vi "Directory handler.vi"() -> ()   [LabVIEW 2011]
panel:
  in  "Type of Files (*.csv; *.txt)":string="Select the Loc"
  in  "Prompt for Directory Diolog":string="Select the Loc"
  out "error in (no error) 2":errorcluster
  out "Path output":path
  in  "Start Path":path
  in  "error in (no error)":errorcluster
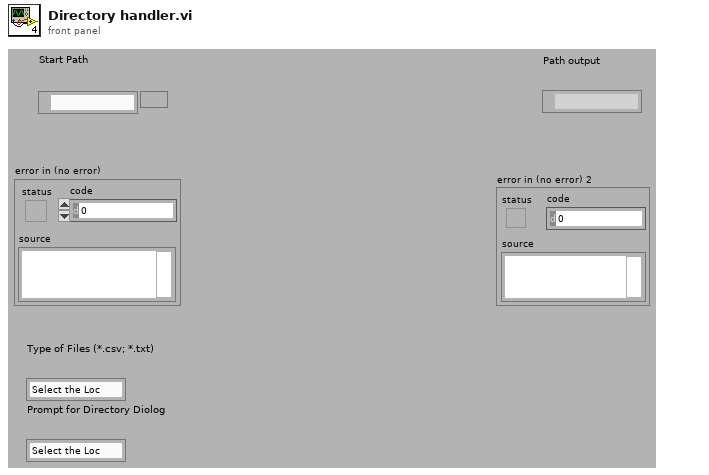
[diagram p1: front panel]
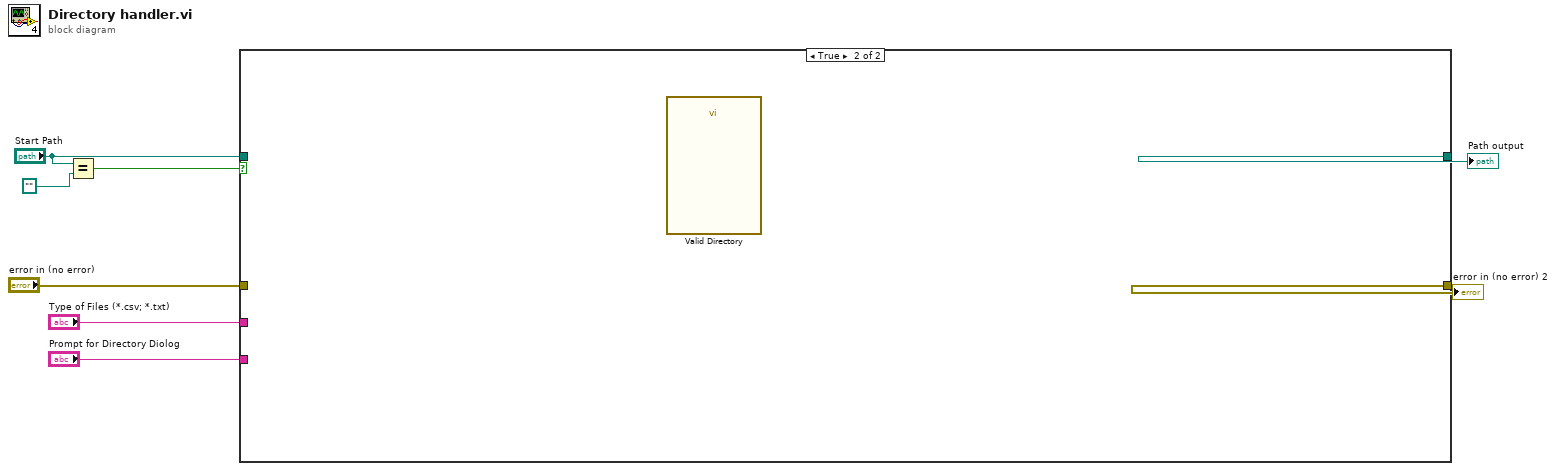
[diagram p0: block diagram]
diagram:
  n1 = Equal?(x="Start Path", y=path "") -> (x = y?=w7:bool)
  n2 = case shown="True" w7 {
    tunnel: "Start Path" -> [w10 _]
    tunnel: [w10 _] -> w5
    tunnel: "error in (no error)" -> [w9 _]
    tunnel: [w9 _] -> w3
    tunnel: "Prompt for Directory Diolog" -> [_ _]
    tunnel: "Type of Files (*.csv; *.txt)" -> [_ _]
    frame False {
    }
    frame True {
      n3 = call "Valid Directory"() -> ()  [unwired: 17 in, 3 out]
    }
  }
  "Path output" <- w5
  "error in (no error) 2" <- w3
